vi "Sweep Step (No Objects).vi"(8 "error in (no error)":errorcluster, 11 "Cluster In":T4={"Field"=0.0, "Rate"=0.0, "Status"={"Sweeping"=FALSE, "Clamped"=FALSE, "Hold"=FALSE, "At Rest"=FALSE, "Quench"=FALSE, "Persistent Mode"=FALSE, "Switch Heater"=FALSE}, "ILM Shut Down?"=FALSE, "IO Info"={"Address"={"Com Port"=1, "ISOBUS Address"=2, "GPIB Address"=24, "Communication"=enum."ISOBUS"}, "Version"=enum."IPS"}, "IO Info (Level Meter)"={"Address"={"Com Port"=1, "ISOBUS Address"=5, "GPIB Address"=24, "Communication"=enum."ISOBUS"}, "ILM Name"="", "Display Channel"=[]}, "Training?"=FALSE, "Training Field and Speed Cluster"={"Training Field"=[0.0, 4.108, 5.78, 8.001], "Training Speed"=[0.0057, 0.0022833333333333334, 0.0011333333333333334, 0.0011333333333333334]}}) -> (0 "error out":errorcluster, 1 "Done?":bool, 2 "field":dbl[unit], 3 "Cluster Out":T4={"Field"=0.0, "Rate"=0.0, "Status"={"Sweeping"=FALSE, "Clamped"=FALSE, "Hold"=FALSE, "At Rest"=FALSE, "Quench"=FALSE, "Persistent Mode"=FALSE, "Switch Heater"=FALSE}, "ILM Shut Down?"=FALSE, "IO Info"={"Address"={"Com Port"=1, "ISOBUS Address"=2, "GPIB Address"=24, "Communication"=enum."ISOBUS"}, "Version"=enum."IPS"}, "IO Info (Level Meter)"={"Address"={"Com Port"=1, "ISOBUS Address"=5, "GPIB Address"=24, "Communication"=enum."ISOBUS"}, "ILM Name"="", "Display Channel"=[]}, "Training?"=FALSE, "Training Field and Speed Cluster"={"Training Field"=[0.0, 4.108, 5.78, 8.001], "Training Speed"=[0.0057, 0.0022833333333333334, 0.0011333333333333334, 0.0011333333333333334]}}, 4 "rate":dbl[unit])   [LabVIEW 2012]
doc: "As the field sweeps, monitor that the current sweep rate is still appropriate and adjust as necessary."
uses:
  Ramping Mode.ctl
  Magnet status.ctl
  Oxford/PSSUBS.LLB/PSIO.ctl
  Oxford/BUSGEN.LLB/OxfordAddress.ctl
  Power Supply.lvclass
panel:
  in  "Ramping Mode":T5
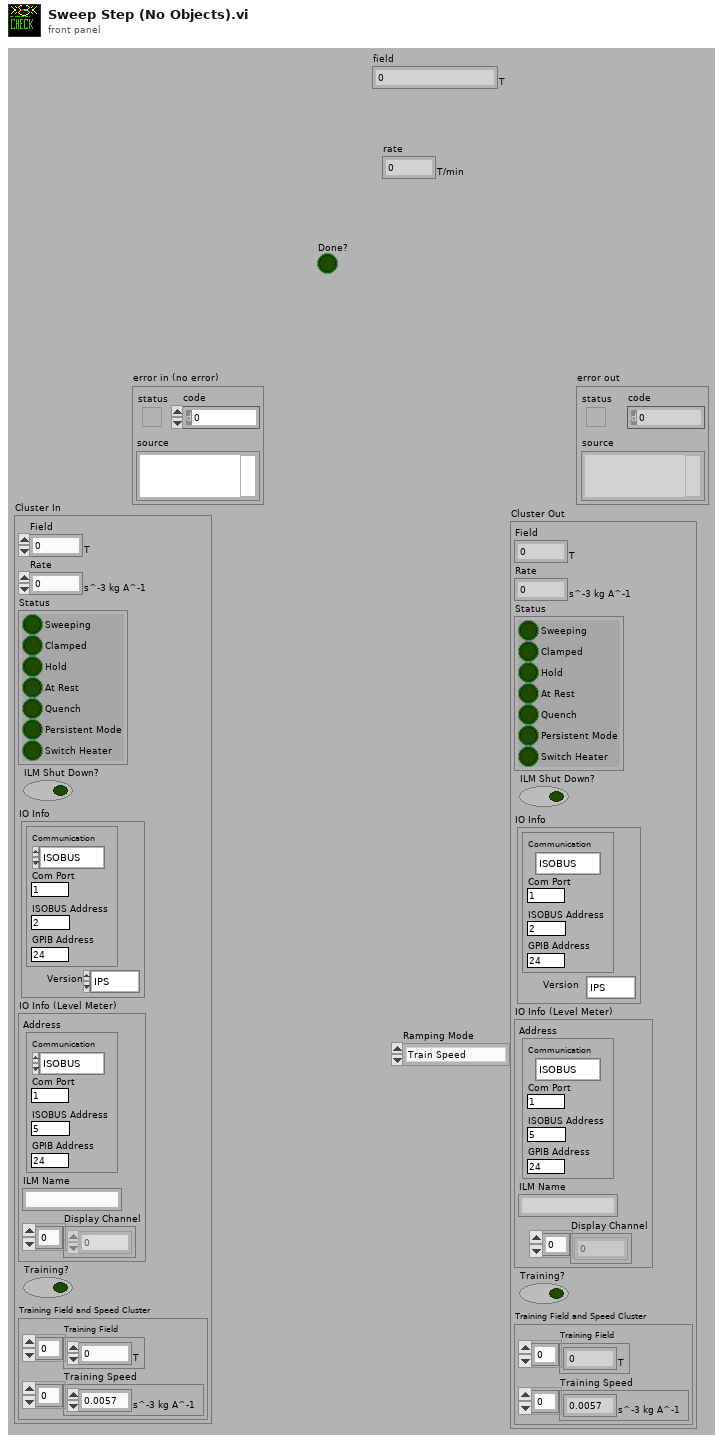
[diagram p1: front panel]
types:
  T1 = typedef "Power Supply.lvclass/Magnet status.ctl" = cluster{"Sweeping":bool, "Clamped":bool, "Hold":bool, "At Rest":bool, "Quench":bool, "Persistent Mode":bool, "Switch Heater":bool}
  T2 = typedef "PSIO.ctl" = cluster{"Address":T3, "Version":enum16{"PS", "IPS"}}
  T3 = typedef "OxfordAddress.ctl" = cluster{"Com Port":i32, "ISOBUS Address":i32, "GPIB Address":i16, "Communication":enum16{"RS232", "ISOBUS", "GPIB", "Gateway"}}
  T4 = cluster{"Field":dbl[unit], "Rate":dbl[unit], "Status":T1, "ILM Shut Down?":bool, "IO Info":T2, "IO Info (Level Meter)":cluster{"Address":T3, "ILM Name":string, "Display Channel":i32[]}, "Training?":bool, "Training Field and Speed Cluster":cluster{"Training Field":dbl[unit][], "Training Speed":dbl[unit][]}}
  T5 = typedef "Power Supply.lvclass/Ramping Mode.ctl" = enum16{"Train Speed", "Maximum Speed", "Manual"}
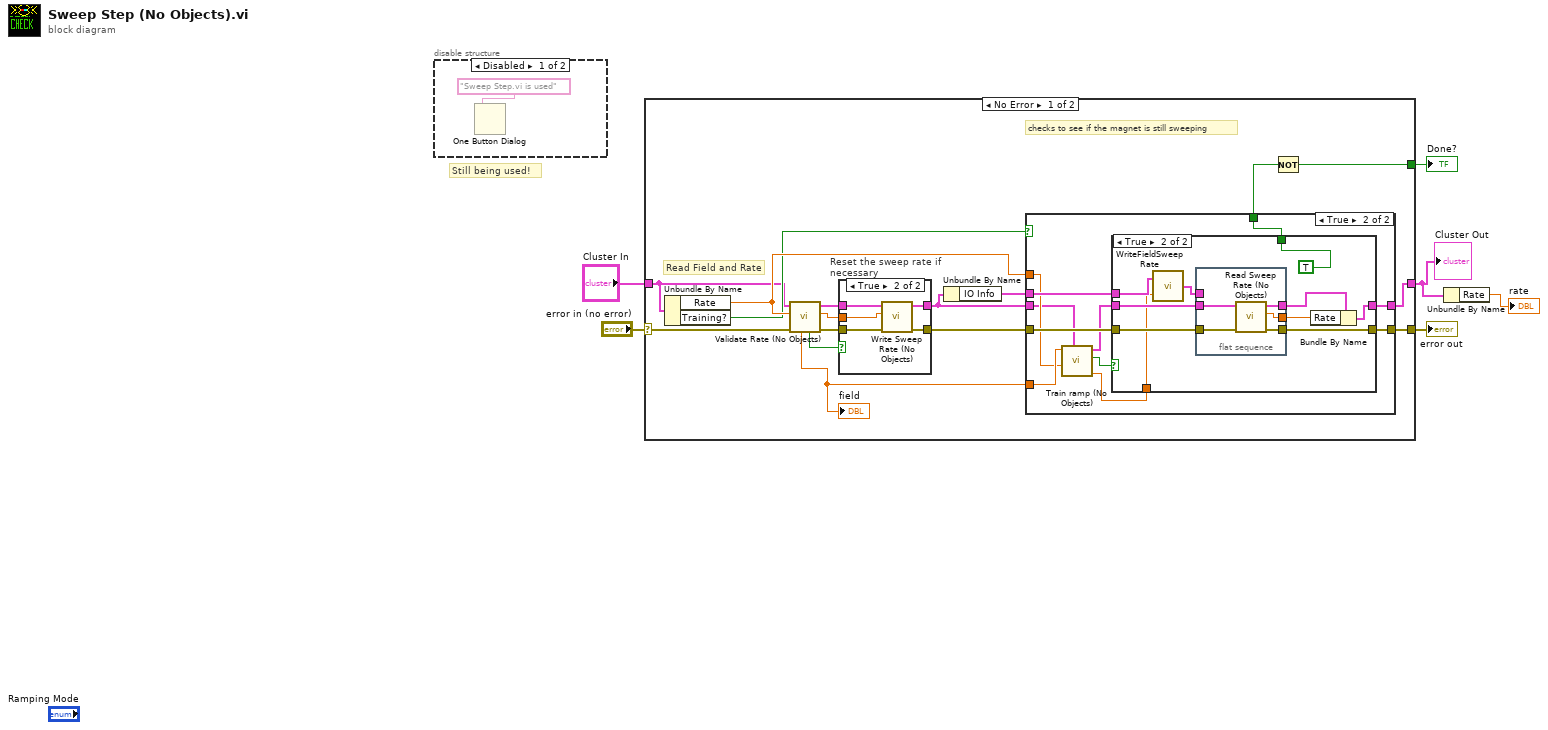
[diagram p0: block diagram]
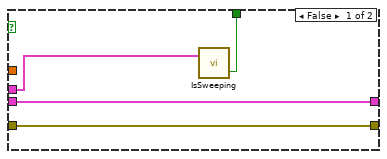
[diagram p3: hidden frame]
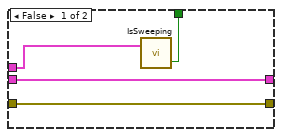
[diagram p4: hidden frame]
diagram:
  # "Still being used!"
  n1 = disable-structure shown="Disabled" {
    frame Disabled {
      n2 = One Button Dialog(message="Sweep Step.vi is used") -> ()  [unwired: 1 in, 1 out]
    }
    frame Enabled {
    }
  }
  n3 = case shown="No Error" "error in (no error)" {
    selector: "error in (no error)" -> [w21 w65]
    tunnel: [w20 _] -> w6
    tunnel: [w18 w65] -> w5
    tunnel: [w14 w66] -> w1
    tunnel: "Cluster In" -> [w8 w66]
    frame No Error {
      # "checks to see if the magnet is still sweeping"
      # "Read Field and Rate"
      n4 = Unbundle By Name(w8) -> ("Rate"=w11:dbl[unit], "Training?"=w10:bool)
      n5 = call "Validate Rate (No Objects).vi"("error IO"=w21, "rate"=w11, "Cluster In"=w8) -> ("error out"=w23:errorcluster, "Coerced rate"=w16:dbl[unit], "Cluster Out"=w22:T4, "Coerced?"=w13:bool, "Field"=w12:dbl[unit])  [unwired: 3 in, 1 out]
      "field" <- w12
      n6 = case "Reset the sweep rate if necessary" shown="True" w13 {
        tunnel: w16 -> [_ w62]
        tunnel: w23 -> [w58 w64]
        tunnel: [w58 w63] -> w19
        tunnel: w22 -> [w59 w60]
        tunnel: [w59 w61] -> w15
        frame False {
        }
        frame True {
          n7 = call "Write Sweep Rate (No Objects).vi"("error in (no error)"=w64, "rate"=w62, "Cluster In"=w60) -> ("error out"=w63:errorcluster, "Cluster Out"=w61:T4)  [unwired: 7 in]
        }
      }
      n8 = Unbundle By Name(w15) -> ("IO Info"=w17:T2)
      n9 = case shown="True" w10 {
        tunnel: w19 -> [w26 w38]
        tunnel: [w26 w37] -> w18
        tunnel: w17 -> [w25 w35]
        tunnel: w15 -> [w27 w28]
        tunnel: [w27 w36] -> w14
        tunnel: w12 -> [_ w30]
        tunnel: w11 -> [_ w29]
        tunnel: [w24 w34] -> w9
        frame False {
          n10 = call "IsSweeping.vi"("IO Info"=w25) -> ("Sweeping"=w24:bool)  [unwired: 2 out]
        }
        frame True {
          n11 = call "Train ramp (No Objects).vi"("Cluster In"=w28, "input"=w29, "field"=w30) -> ("output"=w32:dbl[unit], "change?"=w33:bool, "Cluster Out"=w31:T4)  [unwired: 6 in]
          n12 = case shown="True" w33 {
            tunnel: w38 -> [w41 w50]
            tunnel: [w41 w49] -> w37
            tunnel: w31 -> [w42 w48]
            tunnel: [w42 w47] -> w36
            tunnel: w35 -> [w40 w46]
            tunnel: [w39 TRUE] -> w34
            tunnel: w32 -> [_ w43]
            frame False {
              n13 = call "IsSweeping.vi"("IO Info"=w40) -> ("Sweeping"=w39:bool)  [unwired: 2 out]
            }
            frame True {
              n14 = call "WriteFieldSweepRate.vi"("Sweep rate"=w43, "IO Info"=w46) -> ("IO Info"=w51:T2)
              n15 = flat-sequence {
                tunnel: [w57] -> w45
                tunnel: w48 -> [w53]
                tunnel: [w56] -> w52
                tunnel: w51 -> [_]
                tunnel: w50 -> [w55]
                tunnel: [w54] -> w49
                frame #0 {
                  n16 = call "Read Sweep Rate (No Objects).vi"("error in (no error)"=w55, "Cluster In"=w53) -> ("error out"=w54:errorcluster, "Field sweep rate"=w57:dbl[unit], "Cluster Out"=w56:T4)  [unwired: 7 in]
                }
              }
              n17 = Bundle By Name(cluster=w52, "Rate"=w45) -> (w47:T4)
            }
          }
        }
      }
      n18 = Not(x=w9) -> (.not. x?=w20:bool)
    }
    frame Error {
    }
  }
  "Done?" <- w6
  "error out" <- w5
  "Cluster Out" <- w1
  n19 = Unbundle By Name(w1) -> ("Rate"=→"rate":dbl[unit])
